vi "ATF-Pump-DO array.vi"(7 "Enum":enum16{"Write", "Read"}(ring), 11 "DO Array":bool[](array[boolean])) -> ()   [LabVIEW 2022 SP3]
panel:
  out "DO Array":bool[](array[boolean])
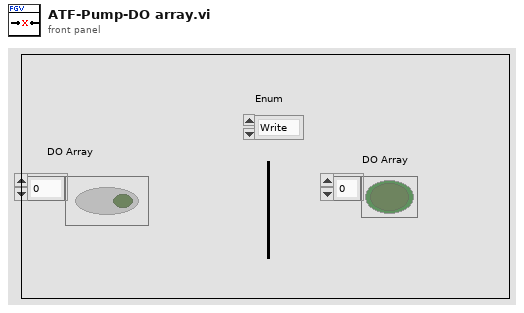
[diagram p1: front panel]
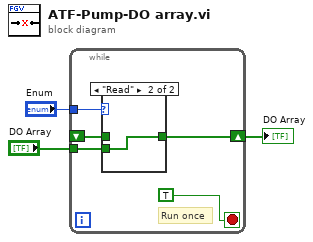
[diagram p0: block diagram]
diagram:
  n1 = while {
    tunnel: "Enum" -> [w7]
    tunnel: "DO Array" -> [w6]
    shift-right: [w5] -> w1
    shift-left: _ -> [w4]
    stop <- TRUE stop-if-true
    # "Run once"
    n2 = case shown="\"Read\"" w7 {
      tunnel: w6 -> [_ w10]
      tunnel: [w9 w10] -> w5
      tunnel: w4 -> [w9 _]
      frame "Write" {
      }
      frame "Read" {
      }
    }
  }
  "DO Array" <- w1
